vi "LDM51全局变量.vi"() -> ()   [LabVIEW 2016, in "LDM51明渠流量计.lvlib"]
panel:
  out "流量计启用":bool[](array[boolean])
  out "总累积流量":dbl
  out "总流量":dbl
  out "平均流速":dbl
  out "平均水位":dbl
  out "累积流量":dbl[](array[numeric])
  out "流速":dbl[](array[numeric])
  out "流量":dbl[](array[numeric])
  out "水位":dbl[](array[numeric])
  out "error out":errorcluster
  out "TX Timestamp":timestamp
  out "TX Data":string
  out "RX Timestamp":timestamp
  out "RX Data":string
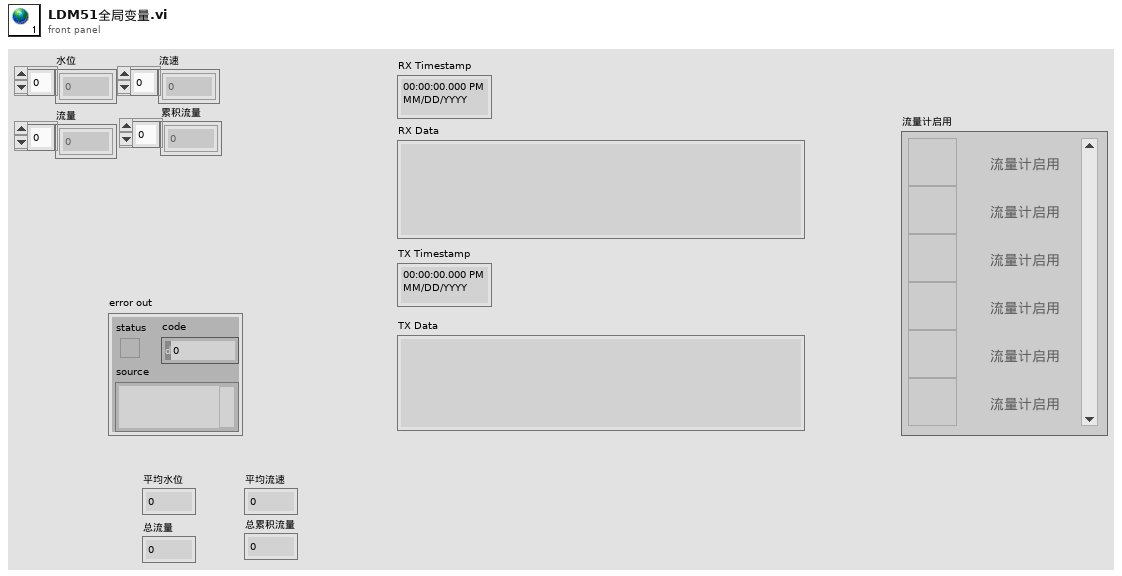
[diagram p1: front panel]
diagram:
